vi "FakeFact3.vi"() -> (0 "error out":errorcluster)   [LabVIEW 2019, in "TestSuiteTestSupport.lvlib" / "FakeLibrary.lvlib"]
uses:
  FakeLibrary.lvlib
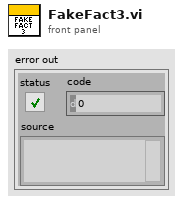
[diagram p1: front panel]
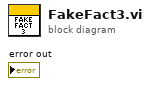
[diagram p0: block diagram]
diagram:
